vi "MessagePrefix.vi"(8 "error in (no error)":errorcluster, 10 "Message in":string, 11 "Logger in":refnum<class "Logger.lvclass">) -> (0 "error out":errorcluster, 2 "Message out":string, 3 "Logger out":refnum<class "Logger.lvclass">)   [LabVIEW 2022 SP3, in "Logger.lvlib" / "Logger.lvclass"]
uses:
  Logger.lvclass
  Logger.lvclass/Logger.ctl
  _MessagePrefixPlaceholder.ctl
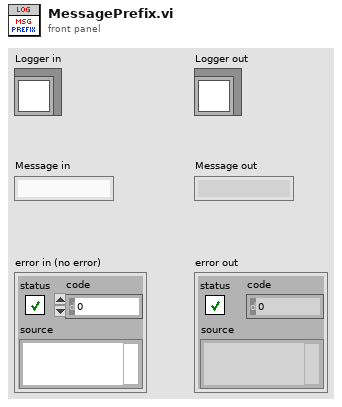
[diagram p1: front panel]
types:
  T1 = typedef "Logger.lvlib/Logger.lvclass/_MessagePrefixPlaceholder.ctl" = enum16{"%sviname", "%lviname"}
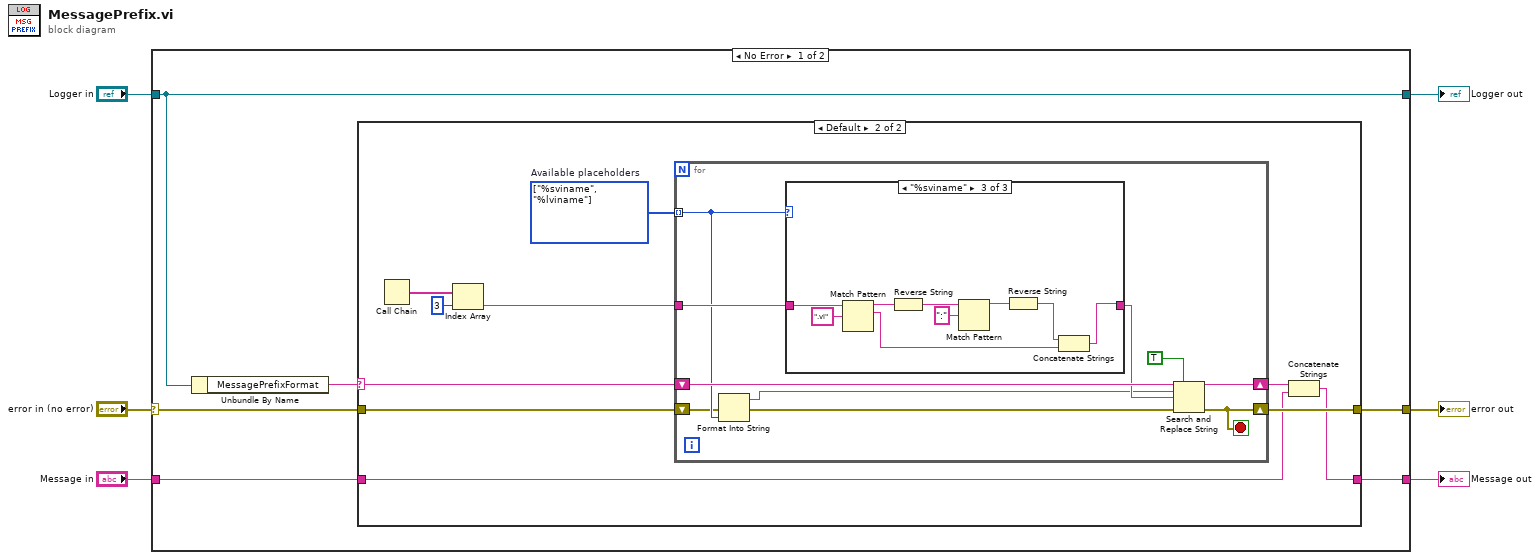
[diagram p0: block diagram]
diagram:
  n1 = case shown="No Error" "error in (no error)" {
    selector: "error in (no error)" -> [w11 w48]
    tunnel: [w10 w48] -> w5
    tunnel: [w12 w47] -> w3
    tunnel: "Logger in" -> [w12 w47]
    tunnel: "Message in" -> [w8 w46]
    tunnel: [w9 w46] -> w1
    frame No Error {
      n2 = Unbundle By Name(w12) -> ("MessagePrefixFormat"=w7:string)
      n3 = case shown="Default" w7 {
        selector: w7 -> [_ w15]
        tunnel: w11 -> [w14 w24]
        tunnel: [w14 w23] -> w10
        tunnel: [w13 w20] -> w9
        tunnel: w8 -> [w13 w19]
        frame "" {
        }
        frame Default {
          w22 = T1[] [enum."%sviname", enum."%lviname"] items=["%sviname", "%lviname"]  # Available placeholders
          n4 = Call Chain() -> (call chain=w18:string[])
          n5 = Index Array(array=w18, index=3) -> (element=w16:string)
          n6 = for {
            shift-right: [w32] -> w23
            shift-left: w24 -> [w26]
            tunnel: w22 -> [w27] mode=indexing
            shift-right: [w31] -> w21
            shift-left: w15 -> [w34]
            tunnel: w16 -> [w30]
            stop <- w32 stop-if-true
            n7 = Format Into String(error in=w26, w27) -> (resulting string=w28:string, error out=w25:errorcluster)  [unwired: 2 in]
            n8 = case shown="\"%sviname\"" w27 {
              tunnel: w30 -> [w35 w36 w40]
              tunnel: [w35 w36 w37] -> w29
              frame Default {
              }
              frame "%lviname" {
              }
              frame "%sviname" {
                n9 = Match Pattern(string=w40, regular expression=".vi") -> (before substring=w44:string, match substring=w39:string)  [unwired: 1 in, 2 out]
                n10 = Reverse String(1:w44) -> (0:w42:string)
                n11 = Match Pattern(string=w42, regular expression=":") -> (before substring=w41:string)  [unwired: 1 in, 3 out]
                n12 = Reverse String(1:w41) -> (0:w38:string)
                n13 = Concatenate Strings(w38, w39) -> (w37:string)
              }
            }
            n14 = Search and Replace String(replace all?=TRUE ("replace all? (F)"), input string=w34, search string=w28, replace string=w29, error in=w25) -> (result string=w31:string, error out=w32:errorcluster)  [unwired: 3 in, 2 out]
          }
          n15 = Concatenate Strings(w21, w19) -> (w20:string)
        }
      }
    }
    frame Error {
    }
  }
  "error out" <- w5
  "Logger out" <- w3
  "Message out" <- w1
